vi "InitEventStream.vi"(8 "error in":errorcluster, 11 "SteamID":string) -> (0 "error out":errorcluster, 3 "EventStreamInfo":T1)   [LabVIEW 2017]
uses:
  Types/SystemEventDataStruct.ctl
  Globals/globals.vi
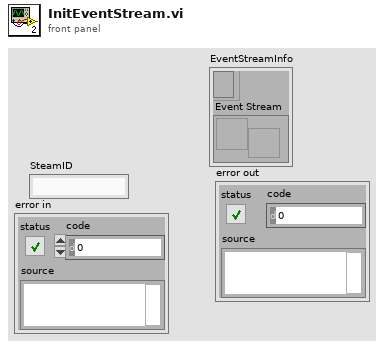
[diagram p1: front panel]
types:
  T1 = cluster{"Event Register":refnum<event-registration>, "Event Stream":refnum<user-event>}
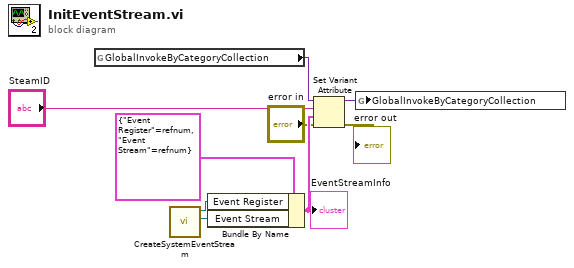
[diagram p0: block diagram]
diagram:
  n1 = global read "globals.vi" "GlobalInvokeByCategoryCollection"() -> (w3:variant)
  n2 = call "CreateSystemEventStream.vi"() -> ("Event Stream Out"=w7:refnum<user-event>, "Event Registration Refnum out"=w6:refnum<event-registration>)  [unwired: 10 in]
  n3 = Bundle By Name(cluster=T1 {"Event Register"=refnum, "Event Stream"=refnum}, "Event Register"=w6, "Event Stream"=w7) -> (w8:T1)
  "EventStreamInfo" <- w8
  n4 = Set Variant Attribute(Variant=w3, name="SteamID", value=w8, error in="error in") -> (Variant out=w4:variant, error out=→"error out":errorcluster)  [unwired: 1 out]
  n5 = global write "globals.vi" "GlobalInvokeByCategoryCollection"(w4) -> ()
